vi "Assign Value.vi"(10 "Assigned Value":refnum<class "Abs_Value.lvclass">, 11 "Value":refnum<class "Abs_Value.lvclass">) -> (3 "Node Out":refnum<class "bt_Node.lvclass">)   [LabVIEW 2021, in "BT.lvlib"]
uses:
  BT.lvlib
  <vilib>/TSA/Abstract Data Classes/Abs_Types/Value/Abs_Value.lvclass
  Support/Nodes/abs_Node/bt_Node.lvclass
  Support/Nodes/Leaves/Assign abs_Value/Assign abs_Value.lvclass
  C:/Users/Tim/Documents/GitHub/LV_Behaviour_Tree/Source/Support/Nodes/abs_Node/bt_Node.lvclass
  Support/Nodes/Leaves/Assign abs_Value/Assign abs_Value.lvclass/Assign abs_Value.ctl
  Support/Nodes/Leaves/Assign abs_Value/Properties/Write Value.vi
  Support/Nodes/Leaves/Assign abs_Value/Properties/Write Assigned Value.vi
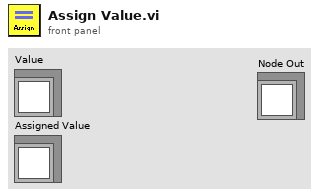
[diagram p1: front panel]
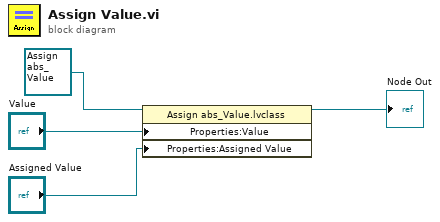
[diagram p0: block diagram]
diagram:
  n1 = property class="Assign abs_Value.lvclass"(reference=refnum<class "Assign abs_Value.lvclass"> refnum ("BT AbsType.lvlib:Assign abs_Value.lvclass"), "Properties:Value"="Value", "Properties:Assigned Value"="Assigned Value") -> (reference out=→"Node Out":refnum<class "Assign abs_Value.lvclass">)  [unwired: 1 in, 1 out]
